vi "Simulation Console.vi"() -> ()   [LabVIEW 2011]
doc: "[Covers: UI1]"
uses:
  Controls/Keypad.xctl
panel:
  in  "Keypad":dbl(xcontrol)
  out "ATM Messages":string
  out "Right Menu 3":string
  out "Right Menu 2":string
  out "Right Menu 1":string
  out "Left Menu 3":string
  out "Left Menu 2":string
  out "Left Menu 1":string
  in  "Right Button 3":bool
  in  "Right Button 2":bool
  in  "Right Button 1":bool
  in  "Left Button 3":bool
  in  "Left Button 2":bool
  in  "Left Button 1":bool
  out "Card Slot":bool
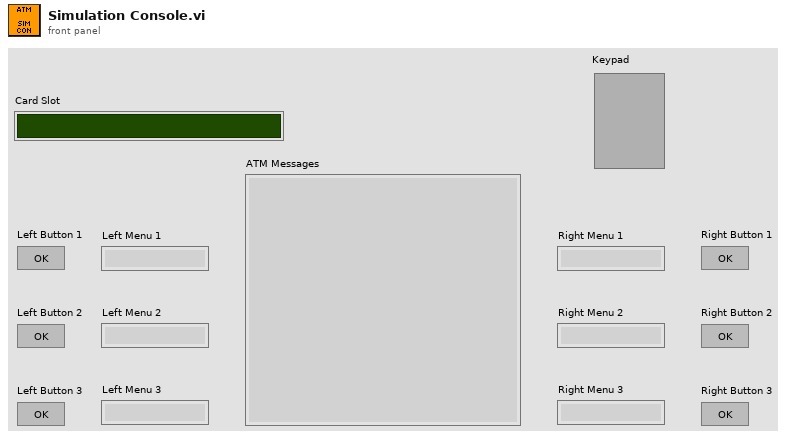
[diagram p1: front panel]
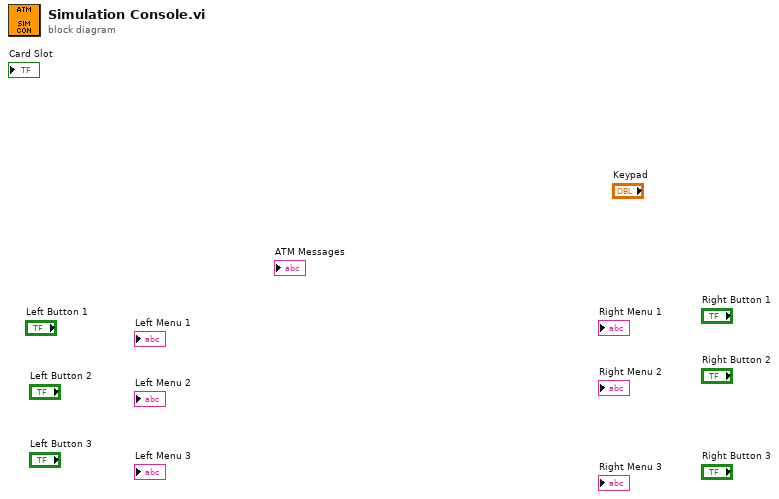
[diagram p0: block diagram]
diagram:
